vi "Series from multiple channels.vi"(8 "Row Numbers":i32[](array[numeric]), 9 "Ordinate Index":i32, 11 "Channel Values":string[][](array[string])) -> (0 "Plot?":bool, 1 "Row Numbers Out":i32[](array[numeric]), 2 "Averaged Values":dbl[](array[numeric]), 3 "Positions":dbl[](array[numeric]))   [LabVIEW 2015]
uses:
  <vilib>/Analysis/baseanly.llb/Mean (DBL).vi
  Results_plotter_Global.vi
  <vilib>/Analysis/NI_AALBase.lvlib
panel:
  out "No of table rows":i32
  out "Number of plot values":i32
  out "Channels":string[](array[string])
  out "element":string
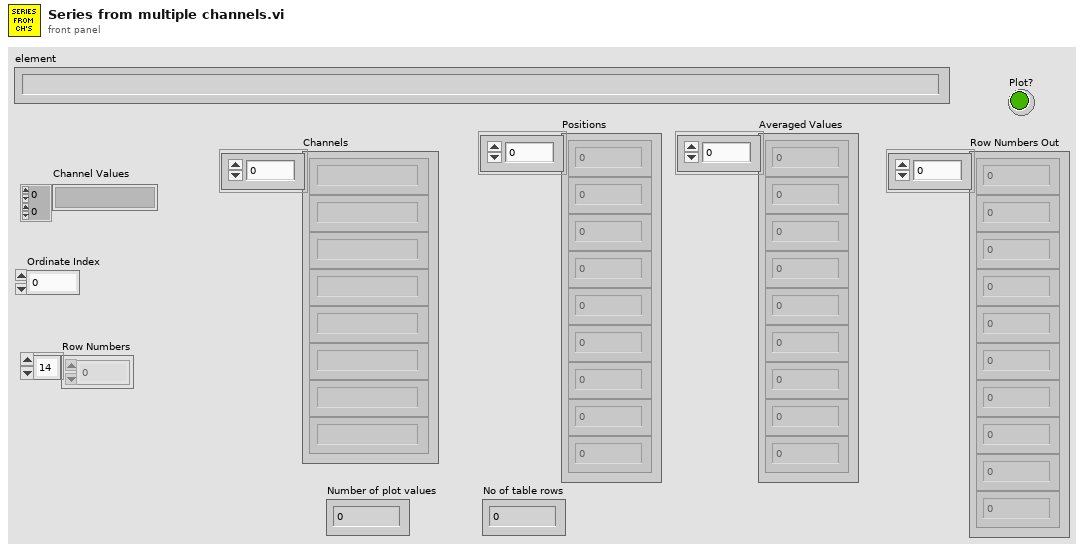
[diagram p1: front panel]
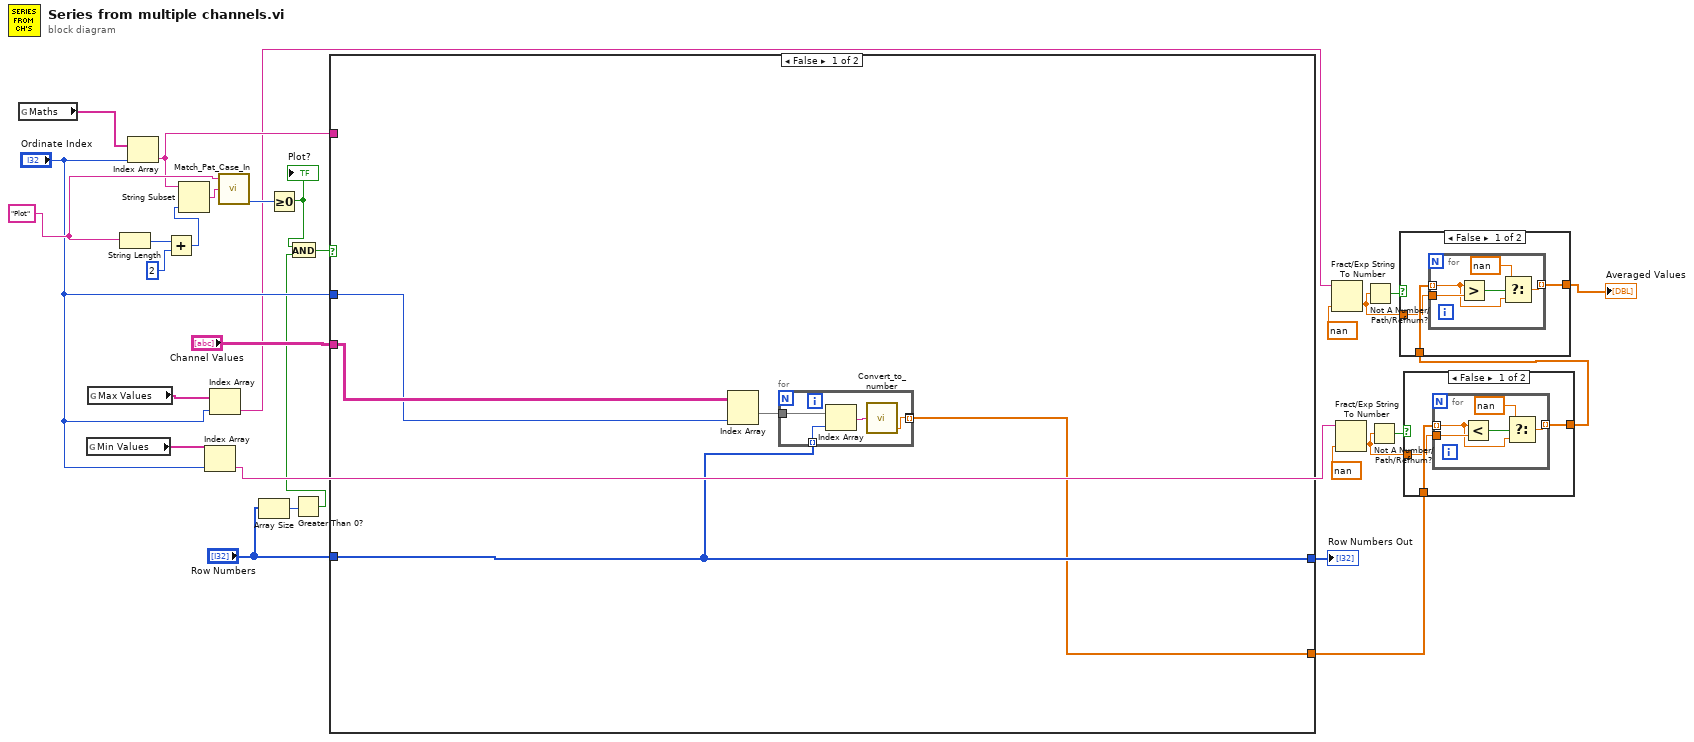
[diagram p0: block diagram]
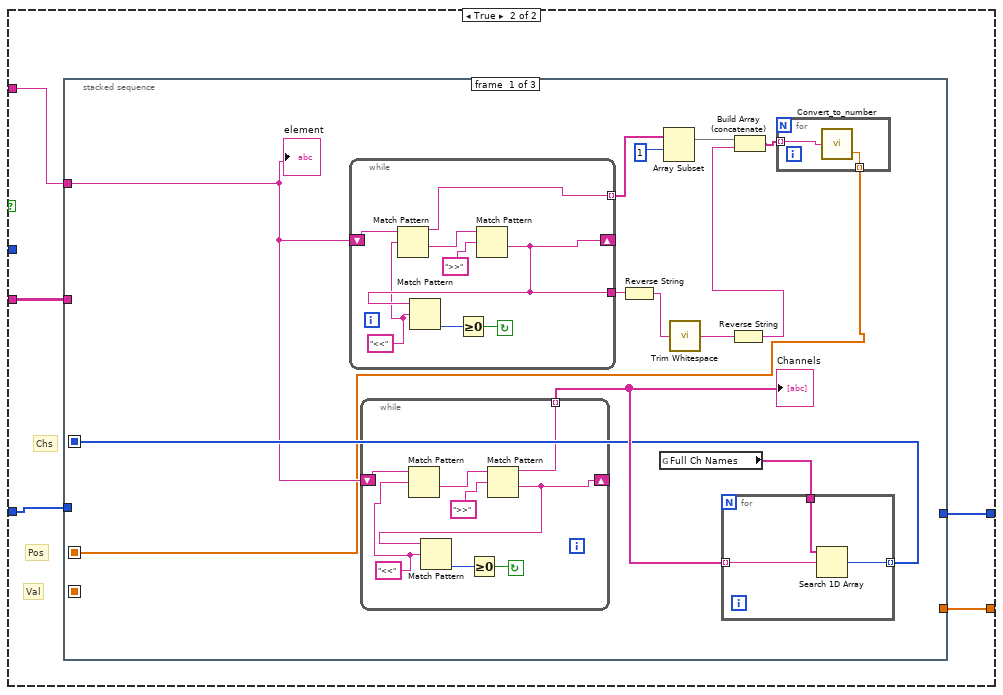
[diagram p4: hidden frame]
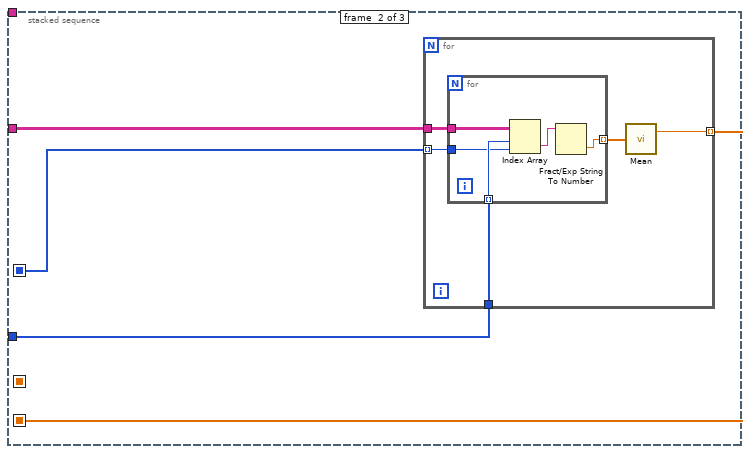
[diagram p5: hidden frame]
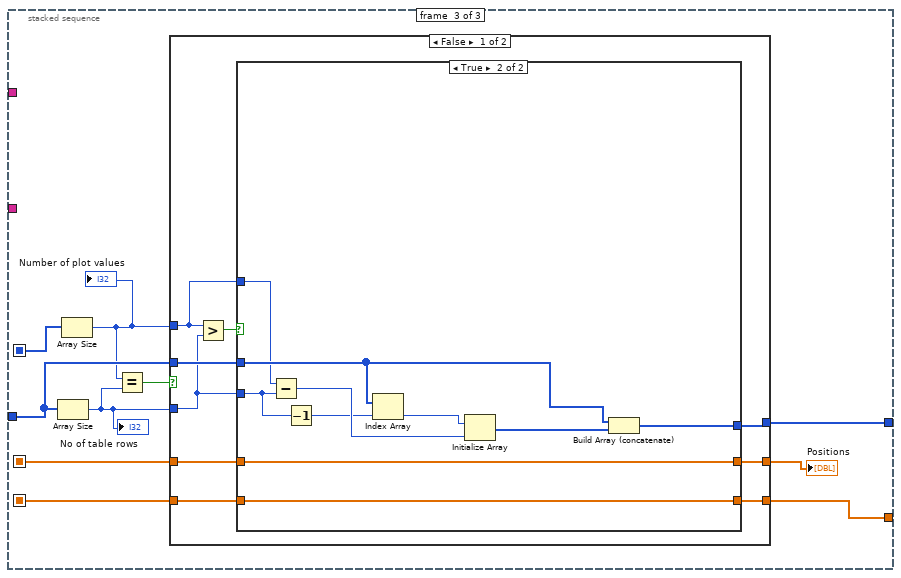
[diagram p6: hidden frame]
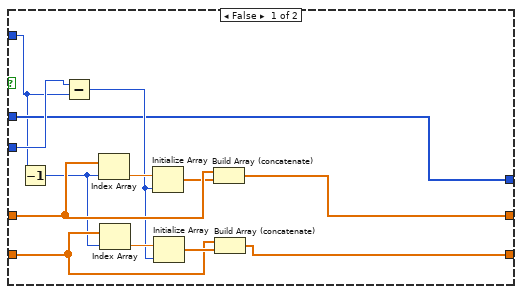
[diagram p7: hidden frame]
diagram:
  w23 = "Plot" ("regular expression")
  n1 = global read "Results_plotter_Global.vi" "Maths"() -> (w24:string[])
  n2 = global read "Results_plotter_Global.vi" "Min Values"() -> (w19:string[])
  n3 = global read "Results_plotter_Global.vi" "Max Values"() -> (w18:string[])
  n4 = String Length(string=w23) -> (length=w26:i32)
  n5 = Index Array(array=w24, index="Ordinate Index") -> (element=w22:string)
  n6 = Add(x=w26, y=2) -> (x+y=w28:i32)
  n7 = String Subset(string=w22, length (rest)=w28) -> (substring=w29:string)  [unwired: 1 in]
  n8 = Index Array(array=w19, index="Ordinate Index") -> (element=w15:string)
  n9 = Index Array(array=w18, index="Ordinate Index") -> (element=w7:string)
  n10 = call "Match_Pat_Case_In.vi"("String to match"=w23, "String"=w29) -> ("offset past match"=w25:i32)  [unwired: 1 in, 3 out]
  n11 = Array Size(array="Row Numbers") -> (size(s)=w2:i32)
  n12 = Greater Or Equal To 0?(x=w25) -> (x >= 0?=w4:bool)
  "Plot?" <- w4
  n13 = Greater Than 0?(x=w2) -> (x > 0?=w1:bool)
  n14 = And(x=w4, y=w1) -> (x .and. y?=w5:bool)
  n15 = case shown="False" w5 {
    tunnel: "Channel Values" -> [w33 w43]
    tunnel: w22 -> [_ w42]
    tunnel: "Row Numbers" -> [w32 w41]
    tunnel: [w32 w40] -> w21
    tunnel: [w31 w39] -> w16
    tunnel: "Ordinate Index" -> [w30 _]
    frame False {
      n16 = Index Array(array=w33, index (col)=w30) -> (element=w34:string[])  [unwired: 1 in]
      n17 = for {
        tunnel: w32 -> [w38] mode=indexing
        tunnel: w34 -> [w37]
        tunnel: [w35] -> w31 mode=indexing
        tunnel: [w35] -> _ mode=indexing
        n18 = Index Array(array=w37, index=w38) -> (element=w36:string)
        n19 = call "Convert_to_number.vi"("string"=w36) -> ("Number"=w35:dbl)  [unwired: 1 out]
      }
    }
    frame True {
      # "Val"
      # "Pos"
      # "Chs"
      n20 = stacked-sequence {
        seq-local: [w47 _ _] -> [_ w80 w101]
        seq-local: [w44 _ _] -> [_ _ w97]
        seq-local: [_ w78 _] -> [_ _ w96]
        tunnel: w43 -> [_ w81 _]
        tunnel: w42 -> [w46 _ _]
        tunnel: w41 -> [_ w79 w98]
        tunnel: [_ _ w99] -> w40
        tunnel: [_ _ w93] -> w39
        frame #0 {
          n21 = while {
            shift-left: w46 -> [w77]
            shift-right: [w72] -> _
            tunnel: [w73] -> w50 mode=indexing
            tunnel: [w72] -> w53
            stop <- w74 continue-if-true
            w71 = "<<" ("regular expression")
            n22 = Match Pattern(string=w77, regular expression=w71) -> (before substring=w73:string, after substring=w76:string)  [unwired: 3 out]
            n23 = Match Pattern(string=w76, regular expression=">>") -> (after substring=w72:string)  [unwired: 4 out]
            n24 = Match Pattern(string=w72, regular expression=w71) -> (offset past match=w75:i32)  [unwired: 4 out]
            n25 = Greater Or Equal To 0?(x=w75) -> (x >= 0?=w74:bool)
          }
          n26 = while {
            tunnel: [w64] -> w48 mode=indexing
            shift-left: w46 -> [w69]
            shift-right: [w67] -> _
            stop <- w65 continue-if-true
            w63 = "<<" ("regular expression")
            n27 = Match Pattern(string=w69, regular expression=w63) -> (after substring=w68:string)  [unwired: 4 out]
            n28 = Match Pattern(string=w68, regular expression=">>") -> (before substring=w64:string, after substring=w67:string)  [unwired: 3 out]
            n29 = Match Pattern(string=w67, regular expression=w63) -> (offset past match=w66:i32)  [unwired: 4 out]
            n30 = Greater Or Equal To 0?(x=w66) -> (x >= 0?=w65:bool)
          }
          "Channels" <- w48
          n31 = Reverse String(1:w53) -> (0:w54:string)
          n32 = global read "Results_plotter_Global.vi" "Full Ch Names"() -> (w49:string[])
          n33 = Array Subset(array=w50, index=1) -> (w51:string[])  [unwired: 1 in]
          n34 = call <vilib>:"Trim Whitespace.vi"("string"=w54) -> ("trimmed string"=w55:string)  [unwired: 1 in]
          n35 = for {
            tunnel: w49 -> [w61]
            tunnel: w48 -> [w60] mode=indexing
            tunnel: [w59] -> w47 mode=indexing
            n36 = Search 1D Array(1D array=w61, element=w60) -> (index of element=w59:i32)  [unwired: 1 in]
          }
          n37 = Reverse String(1:w55) -> (0:w56:string)
          n38 = Build Array (concatenate)(w51, w56) -> (w45:string[])
          n39 = for {
            tunnel: w45 -> [w58] mode=indexing
            tunnel: [w57] -> w44 mode=indexing
            n40 = call "Convert_to_number.vi"("string"=w58) -> ("Number"=w57:dbl)  [unwired: 1 out]
          }
          "element" <- w46
        }
        frame #1 {
          n41 = for {
            tunnel: w81 -> [w86]
            tunnel: w79 -> [w85]
            tunnel: w80 -> [w84] mode=indexing
            tunnel: [w82] -> w78 mode=indexing
            n42 = for {
              tunnel: w86 -> [w91]
              tunnel: w85 -> [w90] mode=indexing
              tunnel: w84 -> [w89]
              tunnel: [w87] -> w83 mode=indexing
              n43 = Index Array(array=w91, index (row)=w90, index (col)=w89) -> (element=w88:string)
              n44 = Fract/Exp String To Number(string=w88) -> (number=w87:dbl)  [unwired: 3 in, 1 out]
            }
            n45 = call-poly <vilib>:"Mean.vi"("X"=w83) -> ("mean"=w82:dbl)  [unwired: 1 out]
          }
        }
        frame #2 {
          n46 = Array Size(array=w98) -> (size(s)=w94:i32)
          "No of table rows" <- w94
          n47 = Array Size(array=w101) -> (size(s)=w95:i32)
          "Number of plot values" <- w95
          n48 = Equal?(x=w95, y=w94) -> (x = y?=w100:bool)
          n49 = case shown="False" w100 {
            tunnel: [w104 w136] -> w99
            tunnel: w98 -> [w105 w136]
            tunnel: [w109 w135] -> w92
            tunnel: w97 -> [w108 w135]
            tunnel: [w107 w134] -> w93
            tunnel: w96 -> [w106 w134]
            tunnel: w95 -> [w103 _]
            tunnel: w94 -> [w102 _]
            frame False {
              n50 = Greater?(x=w103, y=w102) -> (0:w110:bool)
              n51 = case shown="True" w110 {
                tunnel: [w121 w133] -> w109
                tunnel: w108 -> [w122 w133]
                tunnel: [w114 w132] -> w107
                tunnel: w106 -> [w115 w132]
                tunnel: w105 -> [w113 w130]
                tunnel: [w113 w131] -> w104
                tunnel: w103 -> [w112 w129]
                tunnel: w102 -> [w123 w126]
                frame False {
                  n52 = Decrement(x=w112) -> (x-1=w111:i32)
                  n53 = Subtract(x=w123, y=w112) -> (x-y=w116:i32)
                  n54 = Index Array(array=w122, index=w111) -> (element=w119:dbl)
                  n55 = Index Array(array=w115, index=w111) -> (element=w118:dbl)
                  n56 = Initialize Array(w119, w116) -> (w120:dbl[])
                  n57 = Initialize Array(w118, w116) -> (w117:dbl[])
                  n58 = Build Array (concatenate)(w122, w120) -> (w121:dbl[])
                  n59 = Build Array (concatenate)(w115, w117) -> (w114:dbl[])
                }
                frame True {
                  n60 = Subtract(x=w129, y=w126) -> (x-y=w125:i32)
                  n61 = Decrement(x=w126) -> (x-1=w124:i32)
                  n62 = Index Array(array=w130, index=w124) -> (element=w128:i32)
                  n63 = Initialize Array(w128, w125) -> (w127:i32[])
                  n64 = Build Array (concatenate)(w130, w127) -> (w131:i32[])
                }
              }
            }
            frame True {
            }
          }
          "Positions" <- w92
        }
      }
    }
  }
  "Row Numbers Out" <- w21
  n65 = Fract/Exp String To Number(string=w7, default (0 dbl)=nan ("default (0 DBL)")) -> (number=w11:dbl)  [unwired: 2 in, 1 out]
  n66 = Fract/Exp String To Number(string=w15, default (0 dbl)=nan ("default (0 DBL)")) -> (number=w12:dbl)  [unwired: 2 in, 1 out]
  n67 = Not A Number/Path/Refnum?(number/path/refnum=w11) -> (NaN/Path/Refnum?=w9:bool)
  n68 = Not A Number/Path/Refnum?(number/path/refnum=w12) -> (NaN/Path/Refnum?=w14:bool)
  n69 = case shown="False" w14 {
    tunnel: w16 -> [w139 w145]
    tunnel: [w138 w145] -> w8
    tunnel: w12 -> [w137 _]
    frame False {
      n70 = for {
        tunnel: w137 -> [w144]
        tunnel: w139 -> [w142] mode=indexing
        tunnel: [w140] -> w138 mode=indexing
        n71 = Less?(x=w142, y=w144) -> (x < y?=w143:bool)
        n72 = Select(t=nan, s=w143, f=w142) -> (s? t:f=w140:dbl)
      }
    }
    frame True {
    }
  }
  n73 = case shown="False" w9 {
    tunnel: w8 -> [w148 w154]
    tunnel: [w147 w154] -> w6
    tunnel: w11 -> [w146 _]
    frame False {
      n74 = for {
        tunnel: w146 -> [w153]
        tunnel: w148 -> [w151] mode=indexing
        tunnel: [w149] -> w147 mode=indexing
        n75 = Greater?(x=w151, y=w153) -> (0:w152:bool)
        n76 = Select(t=nan, s=w152, f=w151) -> (s? t:f=w149:dbl)
      }
    }
    frame True {
    }
  }
  "Averaged Values" <- w6
